vi "splash.vi"() -> ()   [LabVIEW 2019]
uses:
  _camera/_camera.lvlibp/_cameraClass/_camera.lvclass
  _stage/_stage.lvlibp/_stageClass/_stage.lvclass
  <vilib>/Utility/LVLibp/NI_PackedLibraryUtility.lvlib
panel:
  in  "Select stage(s)":string[](array[combo])
  in  "#":u16=1
  in  "stage path":path=path "C:/Users/lars/Desktop/TransientAbsorptionDAQ/builds/cameras"
  in  "camera path":path=path "C:/Users/lars/Desktop/TransientAbsorptionDAQ/builds/cameras"
  in  "Select camera":string(combo)
  in  "load with selected":bool
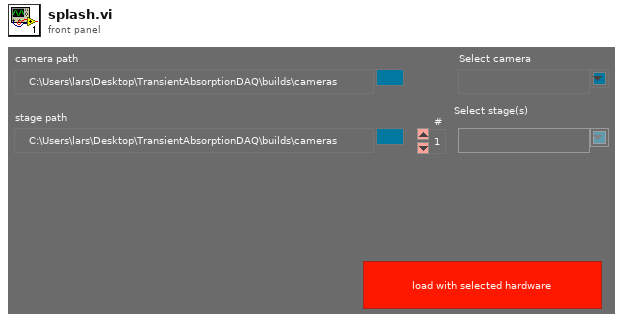
[diagram p1: front panel]
types:
  T1 = enum32{"invalid app kind", "Development System", "Run Time System", "Student Edition", "Embedded LabVIEW", "Evaluation", "Custom"}
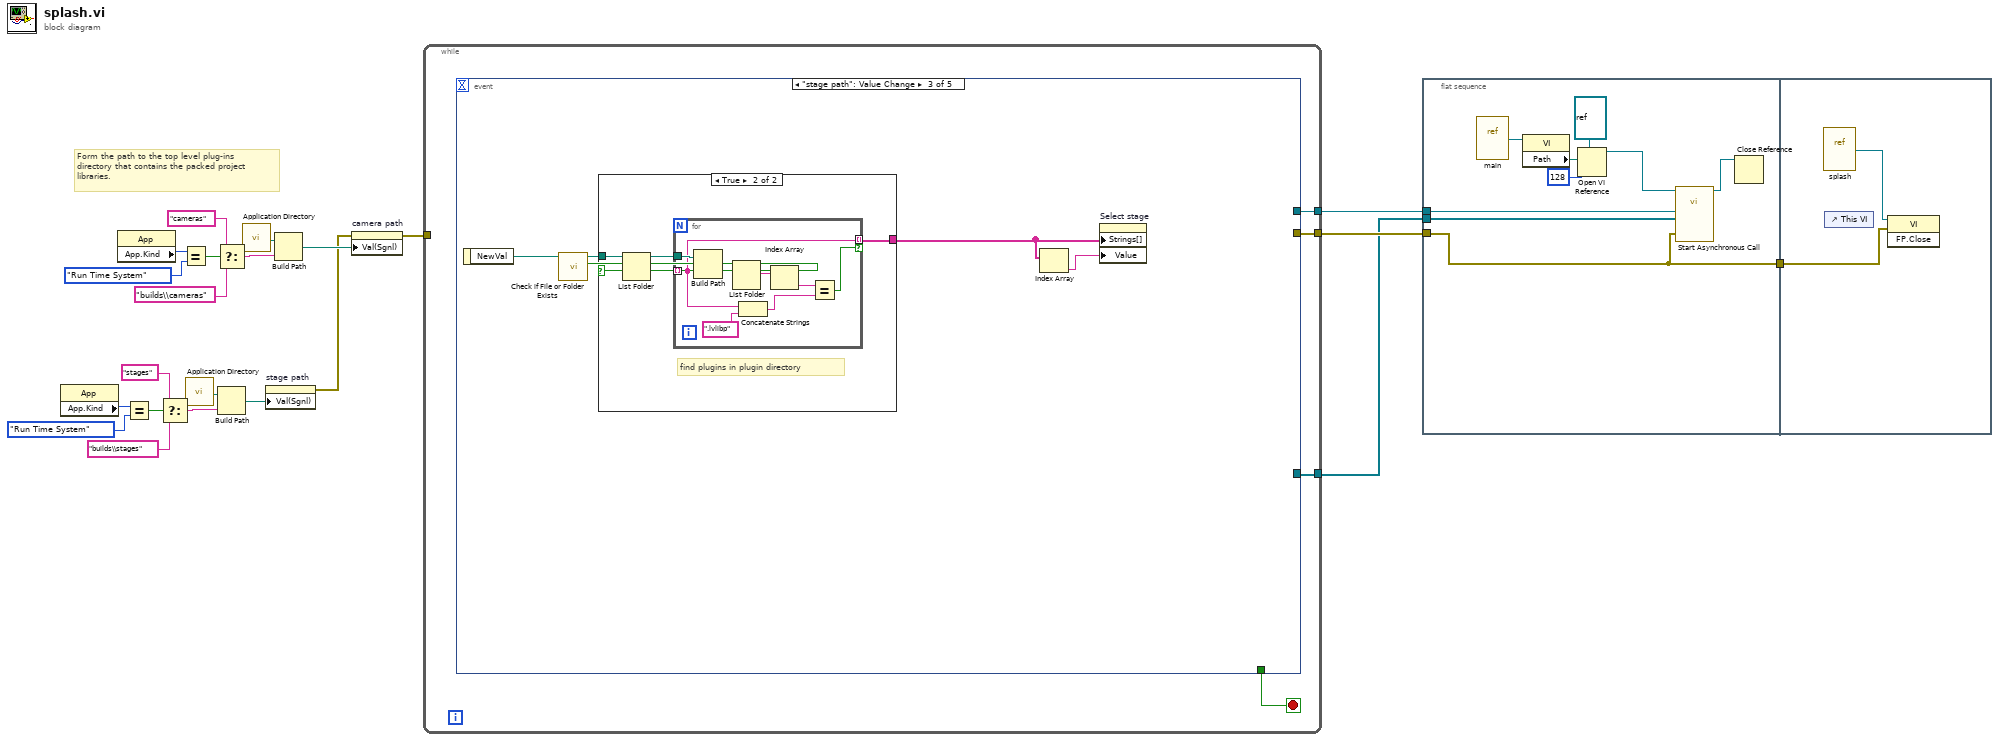
[diagram p0: block diagram]
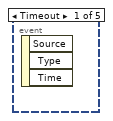
[diagram p2: hidden frame]
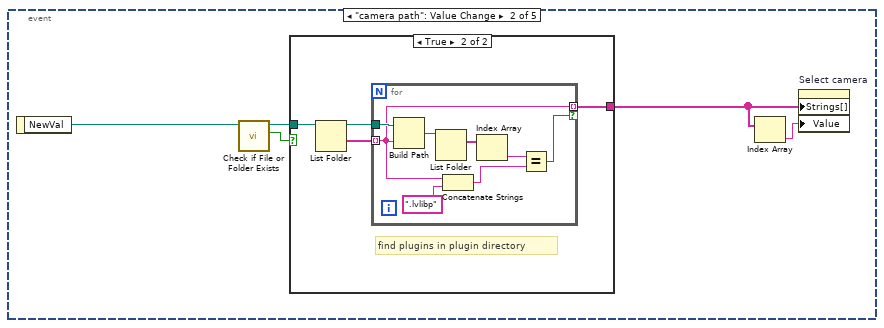
[diagram p3: hidden frame]
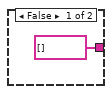
[diagram p4: hidden frame]
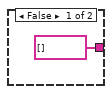
[diagram p5: hidden frame]
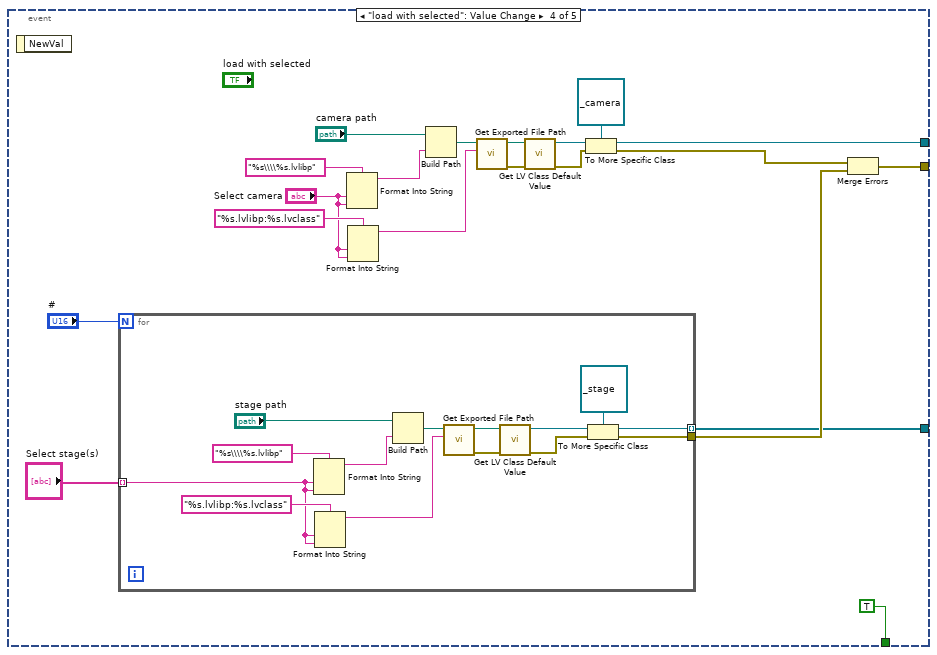
[diagram p6: hidden frame]
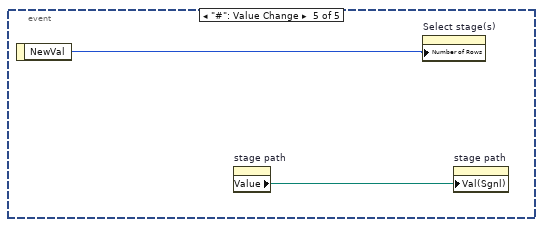
[diagram p7: hidden frame]
diagram:
  # "Form the path to the top level plug-ins\ndirectory that contains the packed project\nlibraries."
  n1 = property class="App"() -> ("App.Kind"=w9:T1)  [unwired: 2 in, 2 out]
  n2 = property class="App"() -> ("App.Kind"=w21:T1)  [unwired: 2 in, 2 out]
  n3 = Equal?(x=w9, y=T1."Run Time System") -> (x = y?=w7:bool)
  n4 = Select(t="stages" ("name or relative path"), s=w7, f="builds\\stages" ("name or relative path")) -> (s? t:f=w4:string)
  n5 = Equal?(x=w21, y=T1."Run Time System") -> (x = y?=w19:bool)
  n6 = call <vilib>:"Application Directory.vi"() -> ("Application Directory"=w10:path)
  n7 = Select(t="cameras" ("name or relative path"), s=w19, f="builds\\cameras" ("name or relative path")) -> (s? t:f=w16:string)
  n8 = Build Path(base path=w10, name or relative path=w4) -> (appended path=w3:path)
  n9 = call <vilib>:"Application Directory.vi"() -> ("Application Directory"=w22:path)
  n10 = property on="stage path" class="Path"("Val(Sgnl)"=w3) -> (error out=w2:errorcluster)  [unwired: 2 in, 1 out]
  n11 = Build Path(base path=w22, name or relative path=w16) -> (appended path=w14:path)
  n12 = property on="camera path" class="Path"(error in=w2, "Val(Sgnl)"=w14) -> (error out=w13:errorcluster)  [unwired: 1 in, 1 out]
  n13 = while {
    tunnel: w13 -> [_]
    tunnel: [w25] -> w15
    tunnel: [w24] -> w12
    tunnel: [w23] -> w1
    stop <- w26 stop-if-true
    n14 = event shown="[2] \"stage path\": Value Change" {
      selector: _ -> [_ _ _ _ _]
      dyn-events: _ -> [_ _ _ _ _]
      timeout: _ -> [_ _ _ _ _]
      tunnel: [_ _ _ TRUE _] -> w26
      tunnel: [_ _ _ w71 _] -> w25
      tunnel: [_ _ _ w66 _] -> w24
      tunnel: [_ _ _ w65 _] -> w23
      event Timeout {
        n15 = event-data() -> ()  [unwired: 1 in, 3 out]
      }
      event "camera path": Value Change {
        n16 = event-data() -> ("NewVal"=w31:path)  [unwired: 1 in]
        n17 = call <vilib>:"Check if File or Folder Exists.vi"("path"=w31) -> ("file or folder exists?"=w30:bool, "dup path"=w29:path)  [unwired: 8 in, 1 out]
        n18 = case shown="True" w30 {
          tunnel: w29 -> [_ w34]
          tunnel: [string[] [] w33] -> w27
          frame False {
          }
          frame True {
            # "find plugins in plugin directory"
            n19 = List Folder(path=w34) -> (path out=w36:path, folder names=w35:string[])  [unwired: 3 in, 2 out]
            n20 = for {
              tunnel: w35 -> [w38] mode=indexing
              tunnel: w36 -> [w44]
              tunnel: [w38] -> w33 mode=indexing if=w37
              n21 = Build Path(base path=w44, name or relative path=w38) -> (appended path=w43:path)
              n22 = List Folder(path=w43) -> (filenames=w42:string[])  [unwired: 3 in, 3 out]
              n23 = Concatenate Strings(w38, ".lvlibp" ("string")) -> (w39:string)
              n24 = Index Array(array=w42) -> (element=w41:string)  [unwired: 1 in]
              n25 = Equal?(x=w41, y=w39) -> (x = y?=w37:bool)
            }
          }
        }
        n26 = Index Array(array=w27) -> (element=w28:string)  [unwired: 1 in]
        n27 = property on="Select camera" class="CmbBox"("Strings[]"=w27, "Value"=w28) -> ()  [unwired: 2 in, 2 out]
      }
      event "stage path": Value Change {
        n28 = event-data() -> ("NewVal"=w47:path)  [unwired: 1 in]
        n29 = call <vilib>:"Check if File or Folder Exists.vi"("path"=w47) -> ("file or folder exists?"=w49:bool, "dup path"=w48:path)  [unwired: 8 in, 1 out]
        n30 = case shown="True" w49 {
          tunnel: w48 -> [_ w52]
          tunnel: [string[] [] w51] -> w46
          frame False {
          }
          frame True {
            # "find plugins in plugin directory"
            n31 = List Folder(path=w52) -> (path out=w54:path, folder names=w53:string[])  [unwired: 3 in, 2 out]
            n32 = for {
              tunnel: w53 -> [w56] mode=indexing
              tunnel: w54 -> [w62]
              tunnel: [w56] -> w51 mode=indexing if=w55
              n33 = Build Path(base path=w62, name or relative path=w56) -> (appended path=w61:path)
              n34 = List Folder(path=w61) -> (filenames=w60:string[])  [unwired: 3 in, 3 out]
              n35 = Concatenate Strings(w56, ".lvlibp" ("string")) -> (w57:string)
              n36 = Index Array(array=w60) -> (element=w59:string)  [unwired: 1 in]
              n37 = Equal?(x=w59, y=w57) -> (x = y?=w55:bool)
            }
          }
        }
        n38 = Index Array(array=w46) -> (element=w45:string)  [unwired: 1 in]
        n39 = property on="Select stage" class="CmbBox"("Strings[]"=w46, "Value"=w45) -> ()  [unwired: 2 in, 2 out]
      }
      event "load with selected": Value Change {
        n40 = event-data() -> ()  [unwired: 1 in, 1 out]
        n41 = for {
          N: "#" -> [_]
          tunnel: [w87] -> w67
          tunnel: [w84] -> w65 mode=indexing
          tunnel: "Select stage(s)" -> [w83] mode=indexing
          n42 = Format Into String(format string="%s\\\\%s.lvlibp", w83, w83) -> (resulting string=w94:string)  [unwired: 2 in, 1 out]
          n43 = Format Into String(format string="%s.lvlibp:%s.lvclass", w83, w83) -> (resulting string=w96:string)  [unwired: 2 in, 1 out]
          n44 = Build Path(base path="stage path", name or relative path=w94) -> (appended path=w95:path)
          n45 = call <vilib>:"Get Exported File Path.vi"("qualified name"=w96, "packed library path"=w95) -> ("error out"=w89:errorcluster, "path"=w88:path)  [unwired: 8 in]
          n46 = call <vilib>:"Get LV Class Default Value.vi"("error in (no error)"=w89, "class path"=w88) -> ("error out"=w90:errorcluster, "object"=w86:refnum<class>)  [unwired: 8 in]
          n47 = To More Specific Class(target class=refnum<class "_stage.lvclass"> refnum ("_stage.lvlibp:_stage.lvclass"), reference=w86, error in=w90) -> (specific class reference=w84:refnum<class "_stage.lvclass">, error out=w87:errorcluster)
        }
        n48 = Format Into String(format string="%s\\\\%s.lvlibp", "Select camera", "Select camera") -> (resulting string=w76:string)  [unwired: 2 in, 1 out]
        n49 = Format Into String(format string="%s.lvlibp:%s.lvclass", "Select camera", "Select camera") -> (resulting string=w79:string)  [unwired: 2 in, 1 out]
        n50 = Build Path(base path="camera path", name or relative path=w76) -> (appended path=w77:path)
        n51 = call <vilib>:"Get Exported File Path.vi"("qualified name"=w79, "packed library path"=w77) -> ("error out"=w81:errorcluster, "path"=w78:path)  [unwired: 8 in]
        n52 = call <vilib>:"Get LV Class Default Value.vi"("error in (no error)"=w81, "class path"=w78) -> ("error out"=w82:errorcluster, "object"=w80:refnum<class>)  [unwired: 8 in]
        n53 = To More Specific Class(target class=refnum<class "_camera.lvclass"> refnum ("_camera.lvlibp:_camera.lvclass"), reference=w80, error in=w82) -> (specific class reference=w71:refnum<class "_camera.lvclass">, error out=w68:errorcluster)
        n54 = Merge Errors(w68, w67) -> (w66:errorcluster)
      }
      event "#": Value Change {
        n55 = event-data() -> ("NewVal"=w97:u16)  [unwired: 1 in]
        n56 = property on="stage path" class="Path"() -> ("Value"=w98:path)  [unwired: 2 in, 2 out]
        n57 = property on="Select stage(s)" class="Arr (strict)"("Number of Rows"=w97) -> ()  [unwired: 2 in, 2 out]
        n58 = property on="stage path" class="Path"("Val(Sgnl)"=w98) -> ()  [unwired: 2 in, 2 out]
      }
    }
  }
  n59 = flat-sequence {
    tunnel: w15 -> [w103]
    tunnel: w12 -> [w101]
    tunnel: [w101] -> w11
    tunnel: w1 -> [w102]
    tunnel: w11 -> [w109]
    frame #0 {
      n60 = vi-ref "main.vi"() -> (w106:refnum<vi>)
      n61 = property class="VI"(reference=w106) -> ("Path"=w105:path)  [unwired: 1 in, 2 out]
      n62 = Open VI Reference(type specifier VI Refnum (for type only)=refnum<vi> refnum, vi path=w105, options=128) -> (vi reference=w104:refnum<vi>)  [unwired: 3 in, 1 out]
      n63 = call-by-ref "Start Asynchronous Call"(reference=w104, "error in (no error)"=w101, "stages"=w102, "_camera"=w103) -> (reference out=w100:refnum<vi>)  [unwired: 10 in, 1 out]
      n64 = Close Reference(reference=w100) -> ()  [unwired: 1 in, 1 out]
    }
    frame #1 {
      n65 = vi-ref "splash.vi"() -> (w108:refnum<vi>)
      n66 = control-ref of="This VI"() -> ()  [unwired: 1 out]
      n67 = invoke class="VI" method="FP.Close"(reference=w108, error in=w109) -> ()  [unwired: 1 in, 3 out]
    }
  }
